vi "Module Identities.vi"(8 "error in (no error)":errorcluster, 11 "Config Monitor Module in":refnum<class "Config Monitor Module.lvclass">) -> (0 "error out":errorcluster, 2 "Identities":refnum<class "Identity.lvclass">[](array[class]), 3 "Config Monitor Module out":refnum<class "Config Monitor Module.lvclass">)   [LabVIEW 2020, in "Volatus.lvlib" / "Config Monitor Module.lvclass"]
uses:
  Config Monitor Module.lvclass
  Identity/Identity.lvclass
  Config Monitor Module.lvclass/Config Monitor Module.ctl
  Config Monitor Identity/Config Monitor Identity.lvclass
  C:/dev/lv20CE/relink/lv-volatus/Volatus/Config Monitor Identity/Config Monitor Identity.lvclass
  C:/dev/lv20CE/relink/lv-volatus/Volatus/Identity/Identity.lvclass
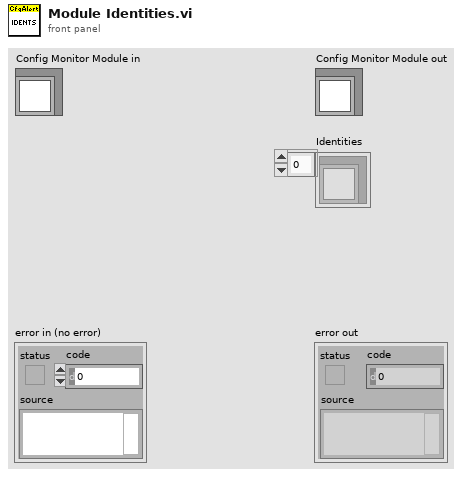
[diagram p1: front panel]
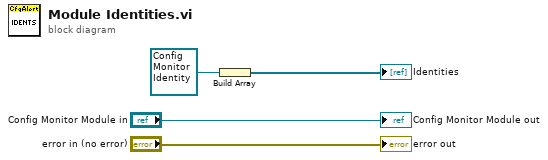
[diagram p0: block diagram]
diagram:
  n1 = Build Array(refnum<class "Config Monitor Identity.lvclass"> refnum ("Volatus:Config Monitor Identity.lvclass")) -> (→"Identities":refnum<class "Config Monitor Identity.lvclass">[])
  "error out" <- "error in (no error)"
  "Config Monitor Module out" <- "Config Monitor Module in"
